vi "Create Cube.vi"() -> (3 "Cube":T1)   [LabVIEW 2020]
uses:
  Controls/Mesh.ctl
  Controls/Triangle.ctl
  Controls/Vector 3D.ctl
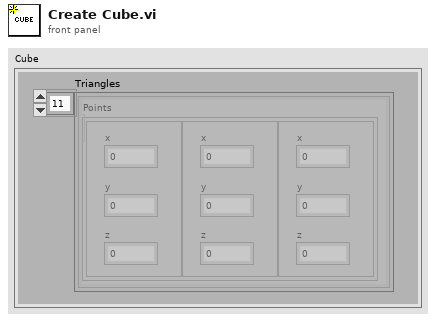
[diagram p1: front panel]
types:
  T1 = typedef "Mesh.ctl" = cluster{"Triangles":T2[]}
  T2 = typedef "Triangle.ctl" = cluster{"Points":T3[]}
  T3 = typedef "Vector 3D.ctl" = cluster{"x":sgl, "y":sgl, "z":sgl}
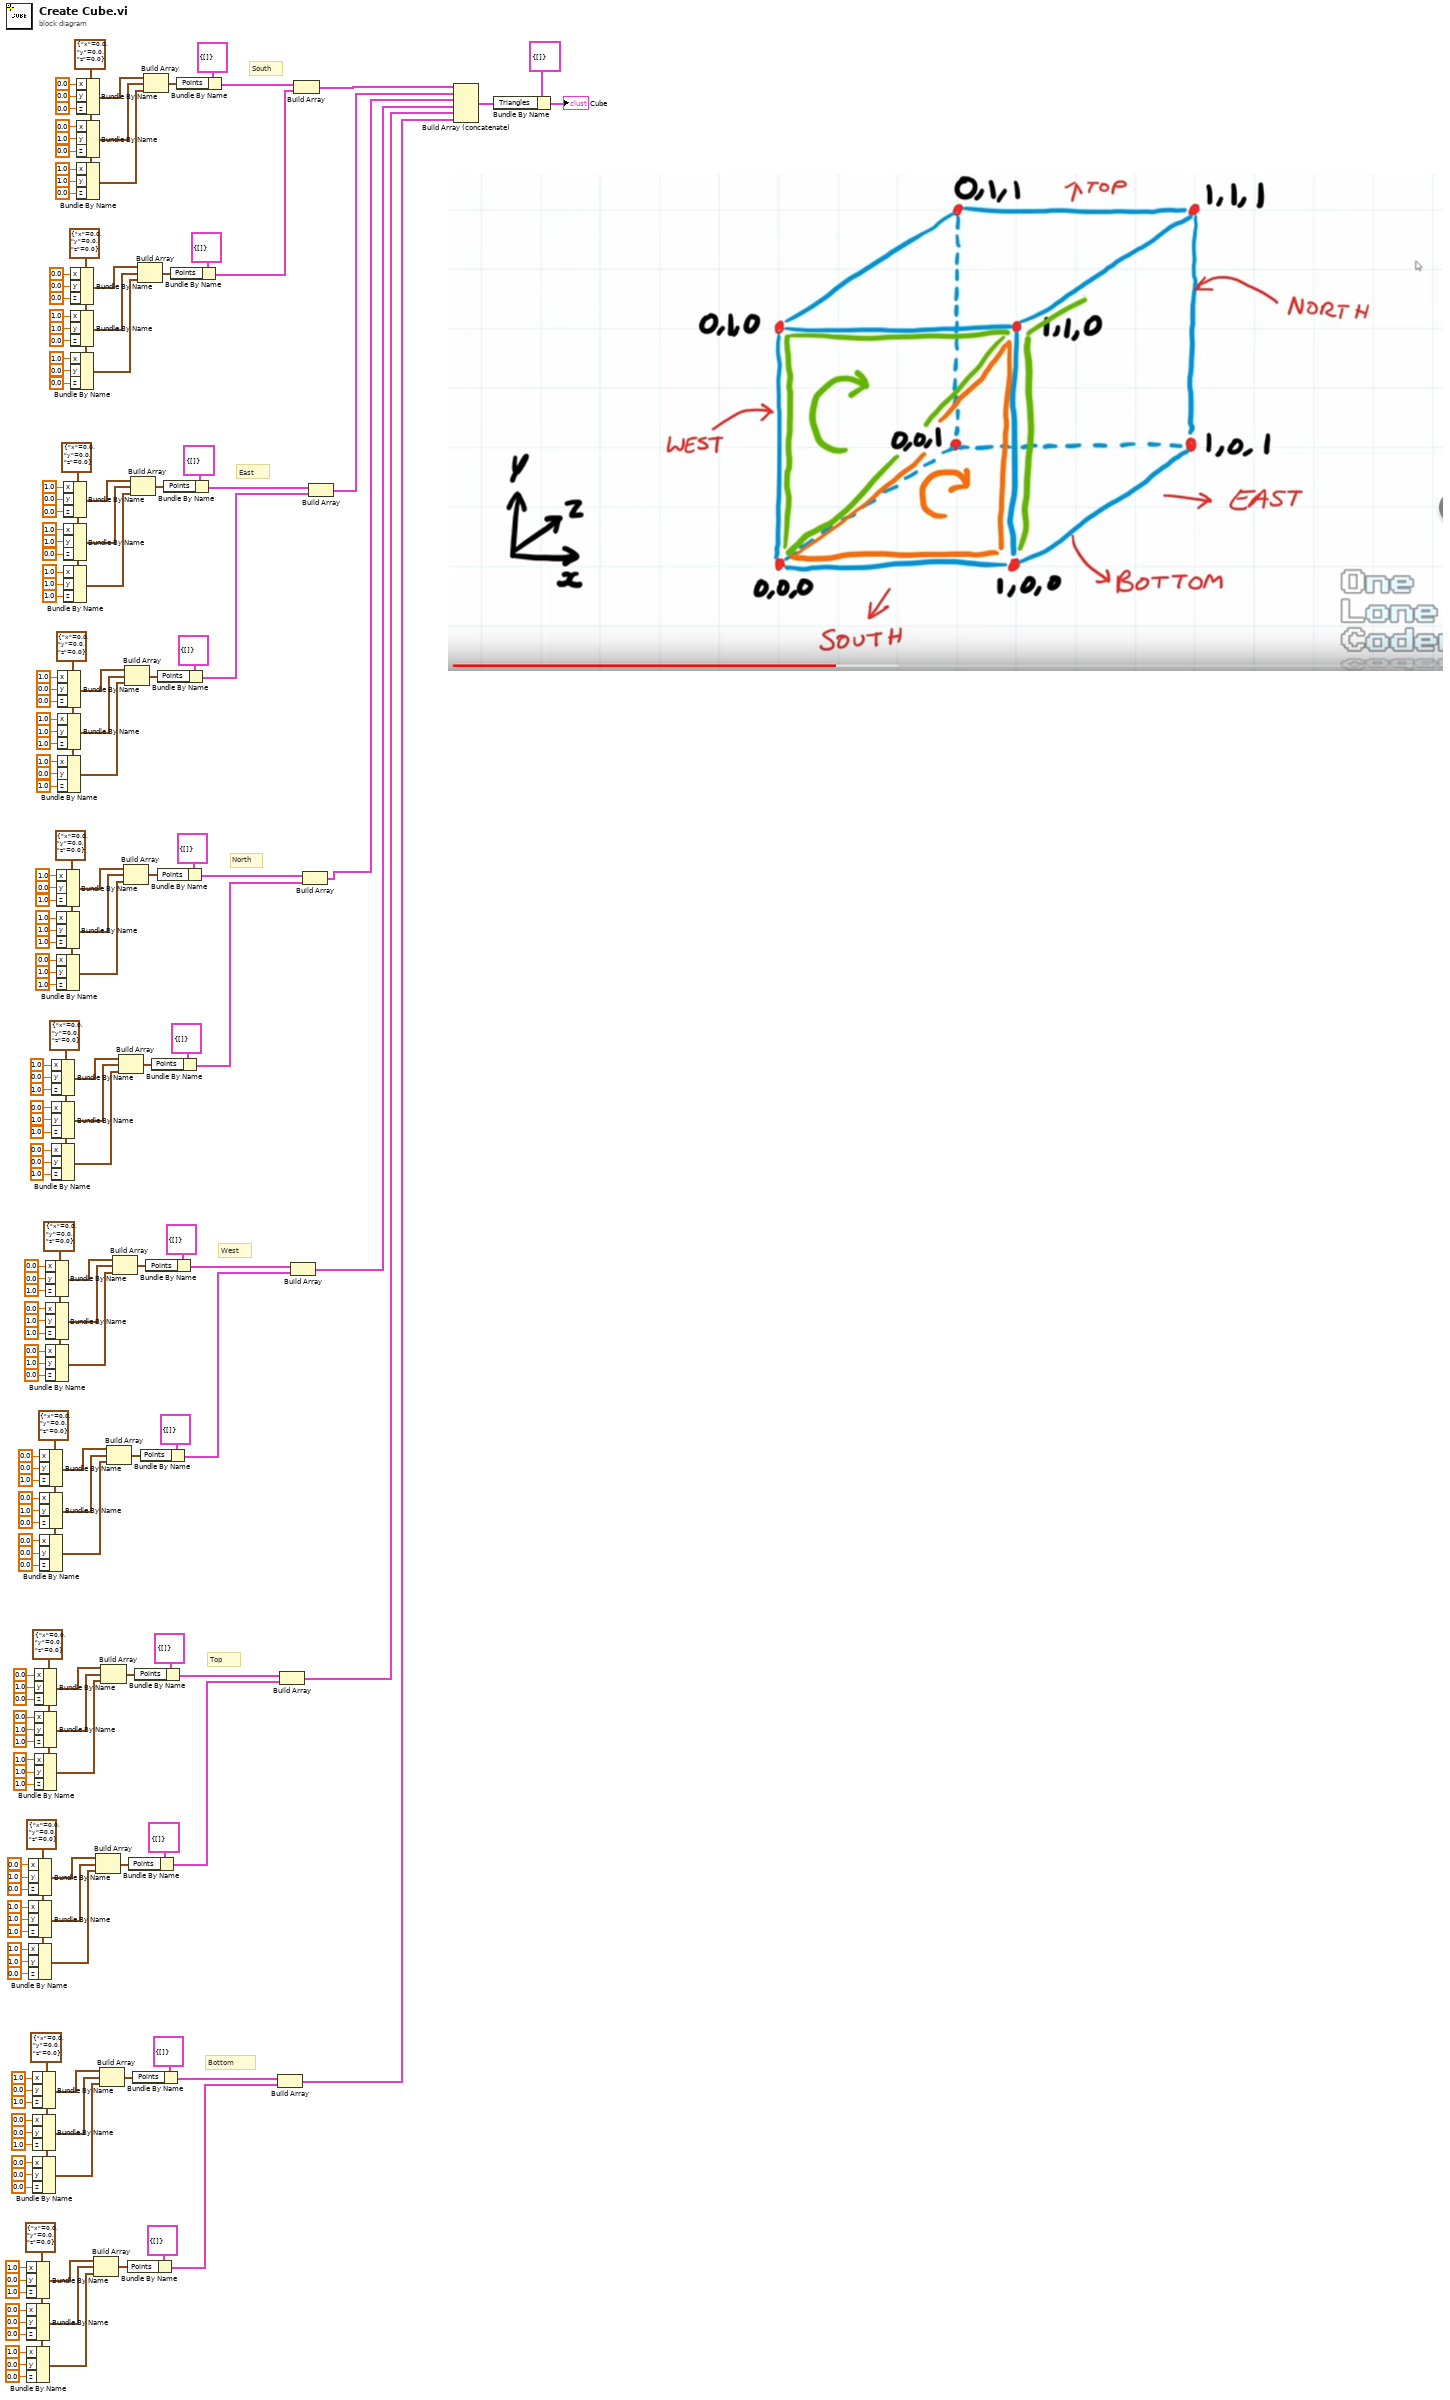
[diagram p0: block diagram]
diagram:
  w27 = T3 {"x"=0.0, "y"=0.0, "z"=0.0} ("Vector 3D")
  w22 = T3 {"x"=0.0, "y"=0.0, "z"=0.0} ("Vector 3D")
  w52 = T3 {"x"=0.0, "y"=0.0, "z"=0.0} ("Vector 3D")
  w57 = T3 {"x"=0.0, "y"=0.0, "z"=0.0} ("Vector 3D")
  w91 = T3 {"x"=0.0, "y"=0.0, "z"=0.0} ("Vector 3D")
  w86 = T3 {"x"=0.0, "y"=0.0, "z"=0.0} ("Vector 3D")
  w116 = T3 {"x"=0.0, "y"=0.0, "z"=0.0} ("Vector 3D")
  w121 = T3 {"x"=0.0, "y"=0.0, "z"=0.0} ("Vector 3D")
  w155 = T3 {"x"=0.0, "y"=0.0, "z"=0.0} ("Vector 3D")
  w150 = T3 {"x"=0.0, "y"=0.0, "z"=0.0} ("Vector 3D")
  w181 = T3 {"x"=0.0, "y"=0.0, "z"=0.0} ("Vector 3D")
  w186 = T3 {"x"=0.0, "y"=0.0, "z"=0.0} ("Vector 3D")
  # "Bottom"
  # "Top"
  # "West"
  # "North"
  # "East"
  # "South"
  n1 = Bundle By Name(cluster=w27, "x"=sgl 1.0, "y"=sgl 0.0, "z"=sgl 1.0) -> (w37:T3)
  n2 = Bundle By Name(cluster=w27, "x"=sgl 0.0, "y"=sgl 0.0, "z"=sgl 0.0) -> (w26:T3)
  n3 = Bundle By Name(cluster=w27, "x"=sgl 1.0, "y"=sgl 0.0, "z"=sgl 0.0) -> (w25:T3)
  n4 = Bundle By Name(cluster=w52, "x"=sgl 0.0, "y"=sgl 1.0, "z"=sgl 0.0) -> (w42:T3)
  n5 = Bundle By Name(cluster=w52, "x"=sgl 1.0, "y"=sgl 1.0, "z"=sgl 1.0) -> (w53:T3)
  n6 = Bundle By Name(cluster=w52, "x"=sgl 1.0, "y"=sgl 1.0, "z"=sgl 0.0) -> (w54:T3)
  n7 = Bundle By Name(cluster=w22, "x"=sgl 1.0, "y"=sgl 0.0, "z"=sgl 1.0) -> (w12:T3)
  n8 = Bundle By Name(cluster=w22, "x"=sgl 0.0, "y"=sgl 0.0, "z"=sgl 1.0) -> (w23:T3)
  n9 = Bundle By Name(cluster=w22, "x"=sgl 0.0, "y"=sgl 0.0, "z"=sgl 0.0) -> (w24:T3)
  n10 = Bundle By Name(cluster=w57, "x"=sgl 0.0, "y"=sgl 1.0, "z"=sgl 0.0) -> (w67:T3)
  n11 = Bundle By Name(cluster=w57, "x"=sgl 0.0, "y"=sgl 1.0, "z"=sgl 1.0) -> (w56:T3)
  n12 = Bundle By Name(cluster=w57, "x"=sgl 1.0, "y"=sgl 1.0, "z"=sgl 1.0) -> (w55:T3)
  n13 = Bundle By Name(cluster=w91, "x"=sgl 0.0, "y"=sgl 0.0, "z"=sgl 1.0) -> (w101:T3)
  n14 = Bundle By Name(cluster=w91, "x"=sgl 0.0, "y"=sgl 1.0, "z"=sgl 0.0) -> (w90:T3)
  n15 = Bundle By Name(cluster=w91, "x"=sgl 0.0, "y"=sgl 0.0, "z"=sgl 0.0) -> (w89:T3)
  n16 = Bundle By Name(cluster=w86, "x"=sgl 0.0, "y"=sgl 0.0, "z"=sgl 1.0) -> (w76:T3)
  n17 = Bundle By Name(cluster=w86, "x"=sgl 0.0, "y"=sgl 1.0, "z"=sgl 1.0) -> (w87:T3)
  n18 = Bundle By Name(cluster=w86, "x"=sgl 0.0, "y"=sgl 1.0, "z"=sgl 0.0) -> (w88:T3)
  n19 = Bundle By Name(cluster=w116, "x"=sgl 1.0, "y"=sgl 0.0, "z"=sgl 1.0) -> (w106:T3)
  n20 = Bundle By Name(cluster=w116, "x"=sgl 0.0, "y"=sgl 1.0, "z"=sgl 1.0) -> (w117:T3)
  n21 = Bundle By Name(cluster=w116, "x"=sgl 0.0, "y"=sgl 0.0, "z"=sgl 1.0) -> (w118:T3)
  n22 = Bundle By Name(cluster=w121, "x"=sgl 1.0, "y"=sgl 0.0, "z"=sgl 1.0) -> (w131:T3)
  n23 = Bundle By Name(cluster=w121, "x"=sgl 1.0, "y"=sgl 1.0, "z"=sgl 1.0) -> (w120:T3)
  n24 = Bundle By Name(cluster=w121, "x"=sgl 0.0, "y"=sgl 1.0, "z"=sgl 1.0) -> (w119:T3)
  n25 = Bundle By Name(cluster=w155, "x"=sgl 1.0, "y"=sgl 0.0, "z"=sgl 0.0) -> (w165:T3)
  n26 = Bundle By Name(cluster=w155, "x"=sgl 1.0, "y"=sgl 1.0, "z"=sgl 1.0) -> (w154:T3)
  n27 = Bundle By Name(cluster=w155, "x"=sgl 1.0, "y"=sgl 0.0, "z"=sgl 1.0) -> (w153:T3)
  n28 = Bundle By Name(cluster=w150, "x"=sgl 1.0, "y"=sgl 0.0, "z"=sgl 0.0) -> (w140:T3)
  n29 = Bundle By Name(cluster=w150, "x"=sgl 1.0, "y"=sgl 1.0, "z"=sgl 0.0) -> (w151:T3)
  n30 = Bundle By Name(cluster=w150, "x"=sgl 1.0, "y"=sgl 1.0, "z"=sgl 1.0) -> (w152:T3)
  n31 = Bundle By Name(cluster=w181, "x"=sgl 0.0, "y"=sgl 0.0, "z"=sgl 0.0) -> (w171:T3)
  n32 = Bundle By Name(cluster=w181, "x"=sgl 1.0, "y"=sgl 1.0, "z"=sgl 0.0) -> (w182:T3)
  n33 = Bundle By Name(cluster=w181, "x"=sgl 1.0, "y"=sgl 0.0, "z"=sgl 0.0) -> (w183:T3)
  n34 = Bundle By Name(cluster=w186, "x"=sgl 0.0, "y"=sgl 0.0, "z"=sgl 0.0) -> (w199:T3)
  n35 = Bundle By Name(cluster=w186, "x"=sgl 0.0, "y"=sgl 1.0, "z"=sgl 0.0) -> (w185:T3)
  n36 = Bundle By Name(cluster=w186, "x"=sgl 1.0, "y"=sgl 1.0, "z"=sgl 0.0) -> (w184:T3)
  n37 = Build Array(w37, w26, w25) -> (w38:T3[])
  n38 = Build Array(w42, w53, w54) -> (w41:T3[])
  n39 = Build Array(w12, w23, w24) -> (w11:T3[])
  n40 = Build Array(w67, w56, w55) -> (w68:T3[])
  n41 = Build Array(w101, w90, w89) -> (w102:T3[])
  n42 = Build Array(w76, w87, w88) -> (w75:T3[])
  n43 = Build Array(w106, w117, w118) -> (w105:T3[])
  n44 = Build Array(w131, w120, w119) -> (w132:T3[])
  n45 = Build Array(w165, w154, w153) -> (w166:T3[])
  n46 = Bundle By Name(cluster=T2 {"Points"=[]} ("Triangle"), "Points"=w38) -> (w8:T2)
  n47 = Bundle By Name(cluster=T2 {"Points"=[]} ("Triangle"), "Points"=w41) -> (w71:T2)
  n48 = Build Array(w140, w151, w152) -> (w139:T3[])
  n49 = Bundle By Name(cluster=T2 {"Points"=[]} ("Triangle"), "Points"=w11) -> (w9:T2)
  n50 = Bundle By Name(cluster=T2 {"Points"=[]} ("Triangle"), "Points"=w68) -> (w70:T2)
  n51 = Build Array(w171, w182, w183) -> (w170:T3[])
  n52 = Bundle By Name(cluster=T2 {"Points"=[]} ("Triangle"), "Points"=w102) -> (w72:T2)
  n53 = Build Array(w199, w185, w184) -> (w200:T3[])
  n54 = Bundle By Name(cluster=T2 {"Points"=[]} ("Triangle"), "Points"=w75) -> (w73:T2)
  n55 = Bundle By Name(cluster=T2 {"Points"=[]} ("Triangle"), "Points"=w105) -> (w135:T2)
  n56 = Bundle By Name(cluster=T2 {"Points"=[]} ("Triangle"), "Points"=w132) -> (w134:T2)
  n57 = Bundle By Name(cluster=T2 {"Points"=[]} ("Triangle"), "Points"=w166) -> (w136:T2)
  n58 = Bundle By Name(cluster=T2 {"Points"=[]} ("Triangle"), "Points"=w139) -> (w137:T2)
  n59 = Bundle By Name(cluster=T2 {"Points"=[]} ("Triangle"), "Points"=w170) -> (w168:T2)
  n60 = Bundle By Name(cluster=T2 {"Points"=[]} ("Triangle"), "Points"=w200) -> (w197:T2)
  n61 = Build Array(w9, w8) -> (w3:T2[])
  n62 = Build Array(w70, w71) -> (w4:T2[])
  n63 = Build Array(w73, w72) -> (w5:T2[])
  n64 = Build Array(w197, w168) -> (w2:T2[])
  n65 = Build Array(w134, w135) -> (w6:T2[])
  n66 = Build Array(w137, w136) -> (w7:T2[])
  n67 = Build Array (concatenate)(w2, w7, w6, w5, w4, w3) -> (w1:T2[])
  n68 = Bundle By Name(cluster=T1 {"Triangles"=[]} ("Mesh"), "Triangles"=w1) -> (→"Cube":T1)
